vi "Get Available 7HP info.vi"(5 "Force Another Read":bool) -> (0 "All Port names":string[](array[string]), 1 "7HP Port names":string[](array[string]), 2 "7HP Serial numbers":string[](array[string]))   [LabVIEW 2020]
uses:
  Controls/Post_Process.ctl
  <vilib>/Instr/_visa.llb/VISA Find Search Mode.ctl
  Globals/Meas_global.vi
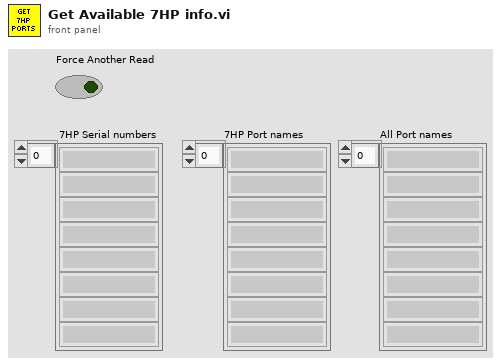
[diagram p1: front panel]
types:
  T1 = typedef "Post_Process.ctl" = enum16{"Take New Data", "Post Process Raw Data File"}
  T2 = typedef "VISA Find Search Mode.ctl" = u32
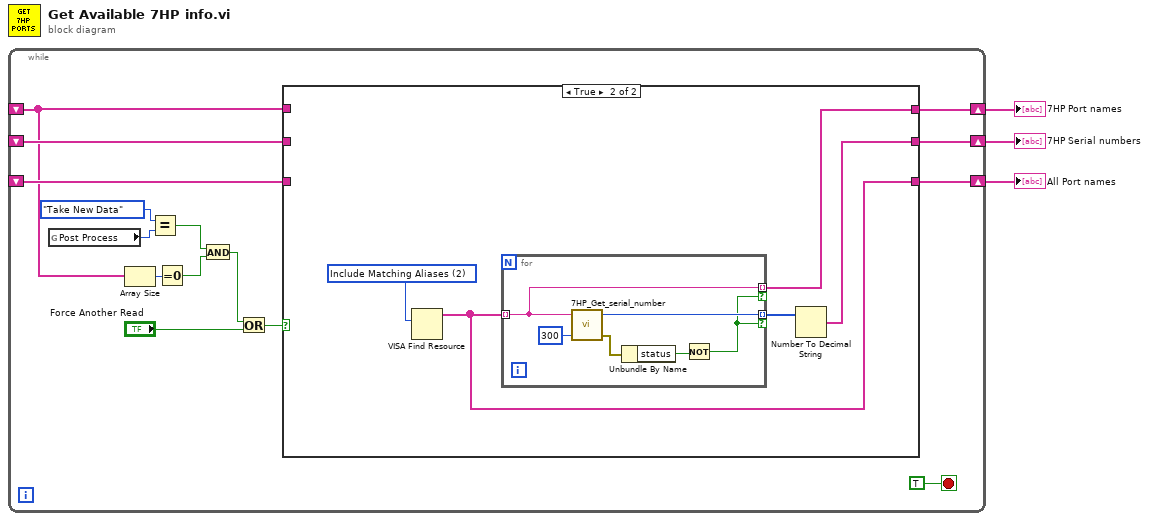
[diagram p0: block diagram]
diagram:
  n1 = while {
    shift-right: [w10] -> w3
    shift-left: _ -> [w4]
    shift-right: [w9] -> w2
    shift-left: _ -> [w7]
    shift-right: [w8] -> w1
    shift-left: _ -> [w6]
    stop <- TRUE stop-if-true
    n2 = global read "Meas_global.vi" "Post Process"() -> (w14:T1)
    n3 = Array Size(array=w4) -> (size(s)=w18:i32)
    n4 = Equal?(x=Post_Process."Take New Data" ("Post Process"), y=w14) -> (x = y?=w12:bool)
    n5 = Equal To 0?(x=w18) -> (x = 0?=w15:bool)
    n6 = And(x=w12, y=w15) -> (x .and. y?=w11:bool)
    n7 = Or(x=w11, y="Force Another Read") -> (x .or. y?=w16:bool)
    n8 = case shown="True" w16 {
      tunnel: [w21 w22] -> w10
      tunnel: [w20 w23] -> w9
      tunnel: [w19 w24] -> w8
      tunnel: w4 -> [w21 _]
      tunnel: w7 -> [w20 _]
      tunnel: w6 -> [w19 _]
      frame False {
      }
      frame True {
        w26 = T2 2 items=["Canonical Names Only"=0, "Aliases Only"=1, "Include Matching Aliases"=2, "Include All Aliases"=4] ("Search Mode")
        n9 = VISA Find Resource(10:w26) -> (3:w24:string[])  [unwired: 2 in, 2 out]
        n10 = for {
          tunnel: w24 -> [w31] mode=indexing
          tunnel: [w32] -> w25 mode=indexing if=w28
          tunnel: [w31] -> w22 mode=indexing if=w28
          n11 = call "7HP_Get_serial_number.vi"("timeout (ms)"=u32 300, "Port"=w31) -> ("Error Out"=w30:errorcluster, "Serial number"=w32:u32)  [unwired: 2 in]
          n12 = Unbundle By Name(w30) -> ("status"=w29:bool)
          n13 = Not(x=w29) -> (.not. x?=w28:bool)
        }
        n14 = Number To Decimal String(number=w25) -> (decimal integer string=w23:string[])  [unwired: 1 in]
      }
    }
  }
  "7HP Port names" <- w3
  "7HP Serial numbers" <- w2
  "All Port names" <- w1
